vi "Default Instrument Setup.vi"(7 "Address":u16, 8 "Error In":errorcluster, 11 "VISA Resource in":refnum<visa-resource-name>) -> (0 "Error Out":errorcluster, 3 "VISA Resource out":refnum<visa-resource-name>)   [LabVIEW 2016, in "KIT QV.lvlib"]
doc: "Sends a default command string to the instrument whenever a new VISA session is opened, or the instrument is reset. Use this VI as a subVI for the <b>Initialize</b> and <b>Reset</b> VIs. Altering this VI could cause these two VIs to operate incorrectly."
uses:
  KIT QV.lvlib
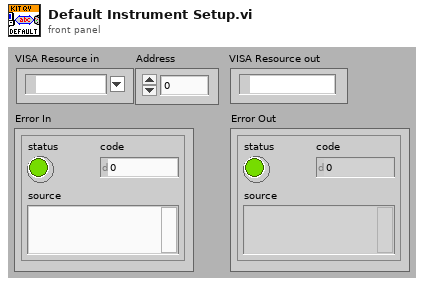
[diagram p1: front panel]
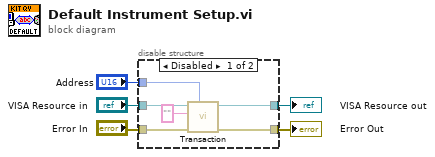
[diagram p0: block diagram]
diagram:
  n1 = disable-structure shown="Disabled" {
    disable-tunnel: "VISA Resource in" -> [w11 w13]
    disable-tunnel: [w10 w13] -> w4
    disable-tunnel: "Error In" -> [w9 w12]
    disable-tunnel: [w8 w12] -> w2
    disable-tunnel: "Address" -> [w6 _]
    frame Disabled {
      n2 = call "Transaction.vi"("Address"=w6, "error in (no error)"=w9, "Command"="" ("Default Setup String"), "VISA Resource in"=w11) -> ("error out"=w8:errorcluster, "VISA Resource out"=w10:refnum<visa-resource-name>)  [unwired: 5 in, 1 out]
    }
    frame Enabled {
    }
  }
  "Error Out" <- w2
  "VISA Resource out" <- w4
